vi "Popup-message.vi"(6 "Message":T1, 10 "Ignore?":bool) -> (2 "Return":bool)   [LabVIEW 2013, in "CameraVision.lvlib" / "CV-UI.lvclass"]
uses:
  CV-UI.lvclass
  Popup-messages.ctl
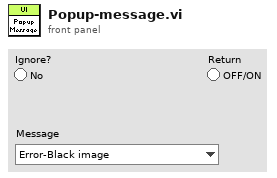
[diagram p1: front panel]
types:
  T1 = typedef "CameraVision.lvlib/CV-UI.lvclass/Popup-messages.ctl" = enum16{"Error-Black image", "Error-Camera config file", "Error-Camera connect", "Error-Grabber init", "Error-Camera setting", "Error-Image offset", "Error-Image import", "Error-Settings file not exist", "Error-Timing source", "Conflict-Filters", "Conflict-Map", "Conflict-Framerate", "Conflict-Charact", "Conflict-Temperature field", "Conflict-Temperature value", "Conflict-Storage-Binary image", "Conflict-Storage-Corrected image", "Conflict-Storage-Map", "Conflict-Storage-Charact", "Conflict-Storage-Temperature field", "Conflict-Storage-Temperature value", "Warning-File exist", "Warning-Parameter reset", "Warning-User cancel", "Info-Images imported"}
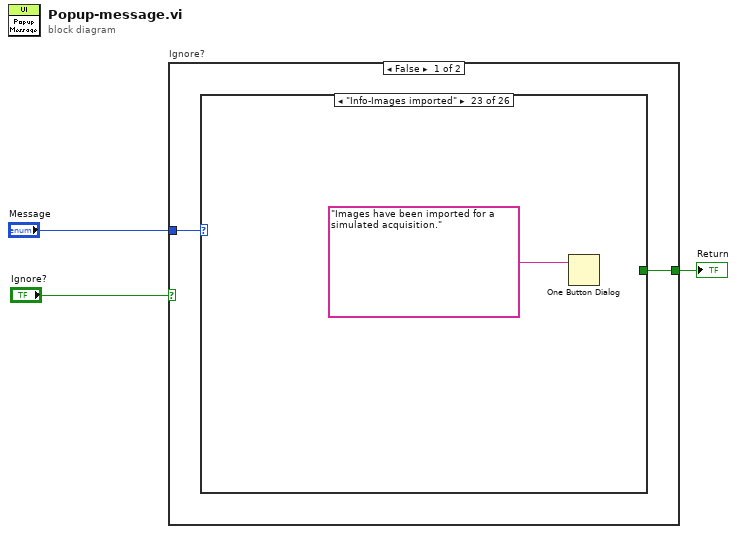
[diagram p0: block diagram]
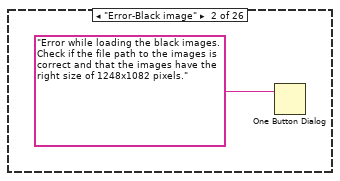
[diagram p3: hidden frame]
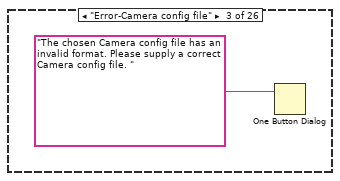
[diagram p4: hidden frame]
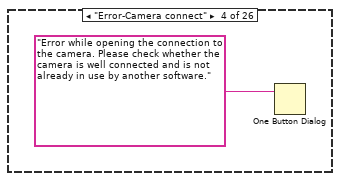
[diagram p5: hidden frame]
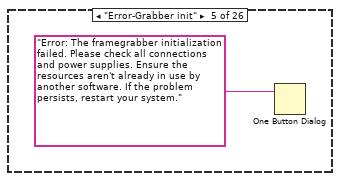
[diagram p6: hidden frame]
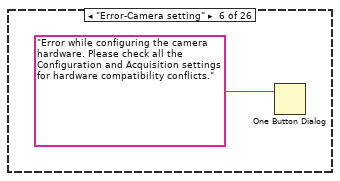
[diagram p7: hidden frame]
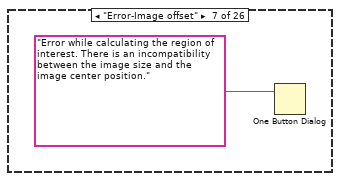
[diagram p8: hidden frame]
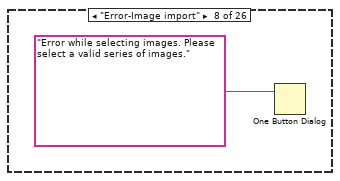
[diagram p9: hidden frame]
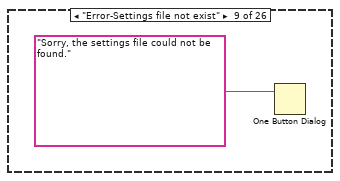
[diagram p10: hidden frame]
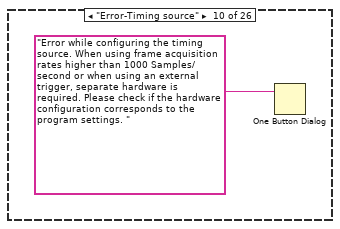
[diagram p11: hidden frame]
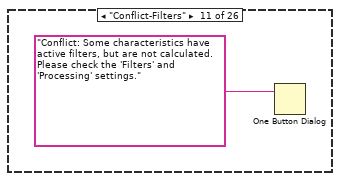
[diagram p12: hidden frame]
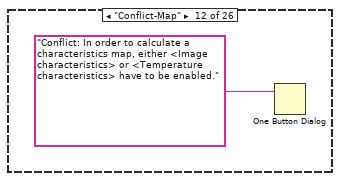
[diagram p13: hidden frame]
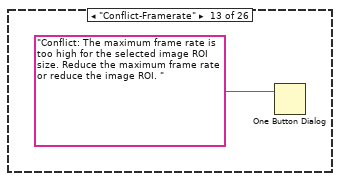
[diagram p14: hidden frame]
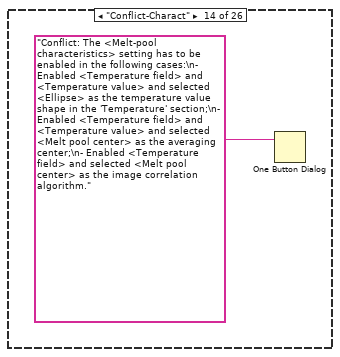
[diagram p15: hidden frame]
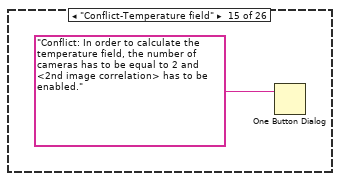
[diagram p16: hidden frame]
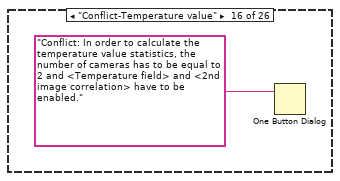
[diagram p17: hidden frame]
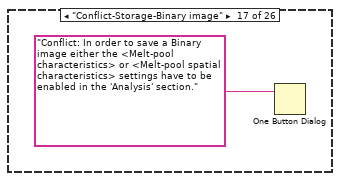
[diagram p18: hidden frame]
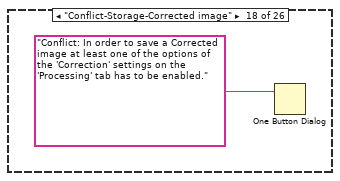
[diagram p19: hidden frame]
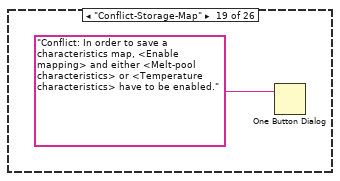
[diagram p20: hidden frame]
diagram:
  n1 = case "Ignore?" shown="False" "Ignore?" {
    tunnel: "Message" -> [w5 _]
    tunnel: [w4 _] -> w1
    frame False {
      n2 = case shown="\"Info-Images imported\"" w5 {
        tunnel: [_ _ _ _ _ _ _ _ _ _ _ _ _ _ _ _ _ _ _ _ _ _ _ _ w29 w33] -> w4
        frame Default {
        }
        frame "Error-Black image" {
          n3 = One Button Dialog(message="Error while loading the black images. Check if the file path to the images is correct and that the images have the right size of 1248x1082 pixels.") -> ()  [unwired: 1 in, 1 out]
        }
        frame "Error-Camera config file" {
          n4 = One Button Dialog(message="The chosen Camera config file has an invalid format. Please supply a correct Camera config file. ") -> ()  [unwired: 1 in, 1 out]
        }
        frame "Error-Camera connect" {
          n5 = One Button Dialog(message="Error while opening the connection to the camera. Please check whether the camera is well connected and is not already in use by another software.") -> ()  [unwired: 1 in, 1 out]
        }
        frame "Error-Grabber init" {
          n6 = One Button Dialog(message="Error: The framegrabber initialization failed. Please check all connections and power supplies. Ensure the resources aren't already in use by another software. If the problem persists, restart your system.") -> ()  [unwired: 1 in, 1 out]
        }
        frame "Error-Camera setting" {
          n7 = One Button Dialog(message="Error while configuring the camera hardware. Please check all the Configuration and Acquisition settings for hardware compatibility conflicts.") -> ()  [unwired: 1 in, 1 out]
        }
        frame "Error-Image offset" {
          n8 = One Button Dialog(message="Error while calculating the region of interest. There is an incompatibility between the image size and the image center position.") -> ()  [unwired: 1 in, 1 out]
        }
        frame "Error-Image import" {
          n9 = One Button Dialog(message="Error while selecting images. Please select a valid series of images.") -> ()  [unwired: 1 in, 1 out]
        }
        frame "Error-Settings file not exist" {
          n10 = One Button Dialog(message="Sorry, the settings file could not be found.") -> ()  [unwired: 1 in, 1 out]
        }
        frame "Error-Timing source" {
          n11 = One Button Dialog(message="Error while configuring the timing source. When using frame acquisition rates higher than 1000 Samples/second or when using an external trigger, separate hardware is required. Please check if the hardware configuration corresponds to the program settings. ") -> ()  [unwired: 1 in, 1 out]
        }
        frame "Conflict-Filters" {
          n12 = One Button Dialog(message="Conflict: Some characteristics have active filters, but are not calculated. Please check the 'Filters' and 'Processing' settings.") -> ()  [unwired: 1 in, 1 out]
        }
        frame "Conflict-Map" {
          n13 = One Button Dialog(message="Conflict: In order to calculate a characteristics map, either <Image characteristics> or <Temperature characteristics> have to be enabled.") -> ()  [unwired: 1 in, 1 out]
        }
        frame "Conflict-Framerate" {
          n14 = One Button Dialog(message="Conflict: The maximum frame rate is too high for the selected image ROI size. Reduce the maximum frame rate or reduce the image ROI. ") -> ()  [unwired: 1 in, 1 out]
        }
        frame "Conflict-Charact" {
          n15 = One Button Dialog(message="Conflict: The <Melt-pool  characteristics> setting has to be enabled in the following cases:\n- Enabled <Temperature field> and <Temperature value> and selected <Ellipse> as the temperature value shape in the 'Temperature' section;\n- Enabled <Temperature field> and <Temperature value> and selected <Melt pool center> as the averaging center;\n- Enabled <Temperature field> and selected <Melt pool center> as the image correlation algorithm.") -> ()  [unwired: 1 in, 1 out]
        }
        frame "Conflict-Temperature field" {
          n16 = One Button Dialog(message="Conflict: In order to calculate the temperature field, the number of cameras has to be equal to 2 and <2nd image correlation> has to be enabled.") -> ()  [unwired: 1 in, 1 out]
        }
        frame "Conflict-Temperature value" {
          n17 = One Button Dialog(message="Conflict: In order to calculate the temperature value statistics, the number of cameras has to be equal to 2 and <Temperature field> and <2nd image correlation> have to be enabled.") -> ()  [unwired: 1 in, 1 out]
        }
        frame "Conflict-Storage-Binary image" {
          n18 = One Button Dialog(message="Conflict: In order to save a Binary image either the <Melt-pool characteristics> or <Melt-pool spatial characteristics> settings have to be enabled in the 'Analysis' section.") -> ()  [unwired: 1 in, 1 out]
        }
        frame "Conflict-Storage-Corrected image" {
          n19 = One Button Dialog(message="Conflict: In order to save a Corrected image at least one of the options of the 'Correction' settings on the 'Processing' tab has to be enabled.") -> ()  [unwired: 1 in, 1 out]
        }
        frame "Conflict-Storage-Map" {
          n20 = One Button Dialog(message="Conflict: In order to save a characteristics map, <Enable mapping> and either <Melt-pool characteristics> or <Temperature characteristics> have to be enabled.") -> ()  [unwired: 1 in, 1 out]
        }
        frame "Conflict-Storage-Charact" {
          n21 = One Button Dialog(message="Conflict: In order to save the  Melt-pool characteristics the corresponding setting has to be enabled in the 'Analysis' section of the 'Processing' tab.") -> ()  [unwired: 1 in, 1 out]
        }
        frame "Conflict-Storage-Temperature field" {
          n22 = One Button Dialog(message="Conflict: In order to save the temperature field, the number of cameras has to be equal to 2 and <Temperature field> and <2nd image correlation> have to be enabled.") -> ()  [unwired: 1 in, 1 out]
        }
        frame "Conflict-Storage-Temperature value" {
          n23 = One Button Dialog(message="Conflict: In order to save the temperature value statistics, the number of cameras has to be equal to 2 and <Temperature field>, <Temperature value> and <2nd image correlation> have to be enabled.") -> ()  [unwired: 1 in, 1 out]
        }
        frame "Info-Images imported" {
          n24 = One Button Dialog(message="Images have been imported for a simulated acquisition.") -> ()  [unwired: 1 in, 1 out]
        }
        frame "Warning-User cancel" {
          n25 = One Button Dialog(message="The operation has been canceled by the user.") -> ()  [unwired: 1 in, 1 out]
        }
        frame "Warning-File exist" {
          n26 = Two Button Dialog(message="A file with the same name already exists. Do you want to Overwrite the existing file anyway or  Cancel the save settings operation?", 1:"Cancel", 2:"Overwrite" ("F button name (\"Cancel\")")) -> (T button?=w29:bool)
        }
        frame "Warning-Parameter reset" {
          n27 = Two Button Dialog(message="Warning: Continuing will overwrite all the user parameters. Do you want to Continue anyway or Cancel the operation?", 1:"Cancel", 2:"Continue" ("F button name (\"Cancel\")")) -> (T button?=w33:bool)
        }
      }
    }
    frame True {
    }
  }
  "Return" <- w1
